vi "AuMT8852B Selected Tests.vi"(5 "Tests (All selected)":T2={"Output power (Selected)"=enum."Output power selected", "Power control (Selected)"=enum."Power control selected", "Modulation index (Selected)"=enum."Modulation index selected", "Initial carrier (Selected)"=enum."Initial carrier selected", "Carrier drift (Selected)"=enum."Carrier drift selected", "Single-slot sensitivity (Selected) "=enum."Single-slot sensitivity selected", "Multi-slot sensitivity (Selected)"=enum."Multi-slot sensitivity selected", "Maximum input power (Selected)"=enum."Maximum input power selected", "Relative transmit power (Selected)"=enum."Rel. transmit power selected", "Carrier frequency stability and modulation (Selected)"=enum."Carrier freq. and stability selected", "Differential phase encoding"=enum."Differential phase selected", "Sensitivity (Selected)"=enum."Sensitivity selected", "BER floor sensitivity (Selected)"=enum."BER floor sensitivity selected", "EDR Maximum input power (Selected)"=enum."EDR Max input power selected"}, 7 "Set/Get (Set)":enum16{"Set", "Get"}(ring), 8 "error in (no error)":errorcluster, 10 "Script (3)":i32=3, 11 "VISA session":refnum<visa-resource-name>) -> (0 "error out":errorcluster, 2 "error code":i32, 3 "VISA session out":refnum<visa-resource-name>, 4 "Tests out":T1={"Output power"=enum."Output power selected", "Power control"=enum."Power control selected", "Modulation index"=enum."Modulation index selected", "Initial carrier"=enum."Initial carrier selected", "Carrier drift"=enum."Carrier drift selected", "Single-slot sensitivity"=enum."Single-slot sensitivity selected", "Multi-slot sensitivity "=enum."Multi-slot sensitivity selected", "Maximum input iower"=enum."Maximum input power selected", "Relative transmit power (Selected)"=enum."Rel. transmit power selected", "Carrier frequency stability and modulation (Selected)"=enum."Carrier freq. and stability selected", "Differential phase encoding"=enum."Differential phase selected", "Sensitivity (Selected)"=enum."Sensitivity selected", "BER floor sensitivity (Selected)"=enum."BER floor sensitivity selected", "EDR Maximum input power (Selected)"=enum."EDR Max input power selected"})   [LabVIEW 2017]
doc: "Anritsu MT8852B Bluetooth Tester\n\nINPUTS\nSet/Get - whether the configuration is being sent to or retrieved from the instrument.\nTests - which tests are selected for the specified script.\n\nOUTPUTS\nTests Out - the present tests selected for the script."
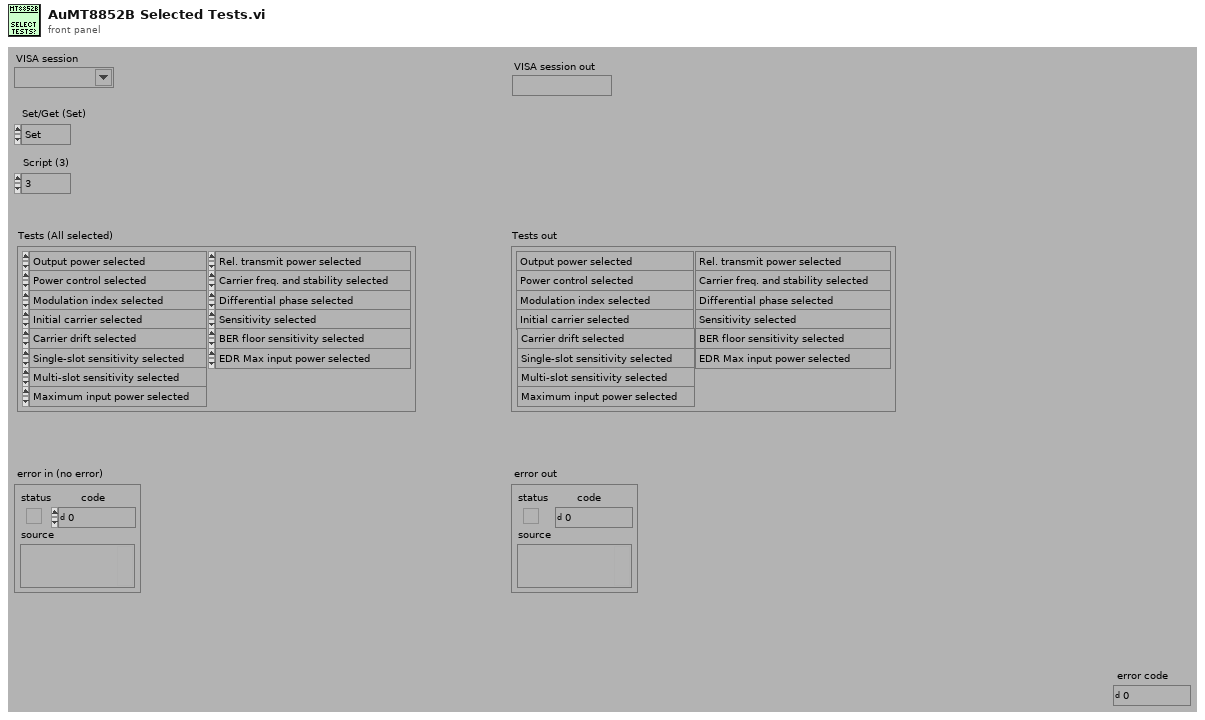
[diagram p1: front panel]
types:
  T1 = cluster{"Output power":enum16{"Output power not selected", "Output power selected"}, "Power control":enum16{"Power control not selected", "Power control selected"}, "Modulation index":enum16{"Modulation index not selected", "Modulation index selected"}, "Initial carrier":enum16{"Initial carrier not selected", "Initial carrier selected"}, "Carrier drift":enum16{"Carrier drift not selected", "Carrier drift selected"}, "Single-slot sensitivity":enum16{"Single-slot sensitivity not selected", "Single-slot sensitivity selected"}, "Multi-slot sensitivity ":enum16{"Multi-slot sensitivity not selected", "Multi-slot sensitivity selected"}, "Maximum input iower":enum16{"Maximum input power not selected", "Maximum input power selected"}, "Relative transmit power (Selected)":enum16{"Rel. transmit power not selected", "Rel. transmit power selected"}, "Carrier frequency stability and modulation (Selected)":enum16{"Carrier freq. and stability not selected", "Carrier freq. and stability selected"}, "Differential phase encoding":enum16{"Differential phase not selected", "Differential phase selected"}, "Sensitivity (Selected)":enum16{"Sensitivity not selected", "Sensitivity selected"}, "BER floor sensitivity (Selected)":enum16{"BER floor sensitivity not selected", "BER floor sensitivity selected"}, "EDR Maximum input power (Selected)":enum16{"EDR Max input power not selected", "EDR Max input power selected"}}
  T2 = cluster{"Output power (Selected)":enum16{"Output power not selected", "Output power selected"}, "Power control (Selected)":enum16{"Power control not selected", "Power control selected"}, "Modulation index (Selected)":enum16{"Modulation index not selected", "Modulation index selected"}, "Initial carrier (Selected)":enum16{"Initial carrier not selected", "Initial carrier selected"}, "Carrier drift (Selected)":enum16{"Carrier drift not selected", "Carrier drift selected"}, "Single-slot sensitivity (Selected) ":enum16{"Single-slot sensitivity not selected", "Single-slot sensitivity selected"}, "Multi-slot sensitivity (Selected)":enum16{"Multi-slot sensitivity not selected", "Multi-slot sensitivity selected"}, "Maximum input power (Selected)":enum16{"Maximum input power not selected", "Maximum input power selected"}, "Relative transmit power (Selected)":enum16{"Rel. transmit power not selected", "Rel. transmit power selected"}, "Carrier frequency stability and modulation (Selected)":enum16{"Carrier freq. and stability not selected", "Carrier freq. and stability selected"}, "Differential phase encoding":enum16{"Differential phase not selected", "Differential phase selected"}, "Sensitivity (Selected)":enum16{"Sensitivity not selected", "Sensitivity selected"}, "BER floor sensitivity (Selected)":enum16{"BER floor sensitivity not selected", "BER floor sensitivity selected"}, "EDR Maximum input power (Selected)":enum16{"EDR Max input power not selected", "EDR Max input power selected"}}
  T3 = enum16{"Simulate", "Range check", "Cache", "Query instrument status"}
  T4 = enum16{"Output power not selected", "Output power selected"}
  T5 = enum16{"Power control not selected", "Power control selected"}
  T6 = enum16{"Modulation index not selected", "Modulation index selected"}
  T7 = enum16{"Initial carrier not selected", "Initial carrier selected"}
  T8 = enum16{"Carrier drift not selected", "Carrier drift selected"}
  T9 = enum16{"Single-slot sensitivity not selected", "Single-slot sensitivity selected"}
  T10 = enum16{"Multi-slot sensitivity not selected", "Multi-slot sensitivity selected"}
  T11 = enum16{"Maximum input power not selected", "Maximum input power selected"}
  T12 = enum16{"Rel. transmit power not selected", "Rel. transmit power selected"}
  T13 = enum16{"Carrier freq. and stability not selected", "Carrier freq. and stability selected"}
  T14 = enum16{"Differential phase not selected", "Differential phase selected"}
  T15 = enum16{"Sensitivity not selected", "Sensitivity selected"}
  T16 = enum16{"BER floor sensitivity not selected", "BER floor sensitivity selected"}
  T17 = enum16{"EDR Max input power not selected", "EDR Max input power selected"}
  T18 = cluster{"[0]":i16, "[1]":i16, "[2]":i16, "[3]":i16, "[4]":i16, "[5]":i16, "[6]":i16, "[7]":i16, "[8]":i16, "[9]":i16, "[10]":i16, "[11]":i16, "[12]":i16, "[13]":i16}
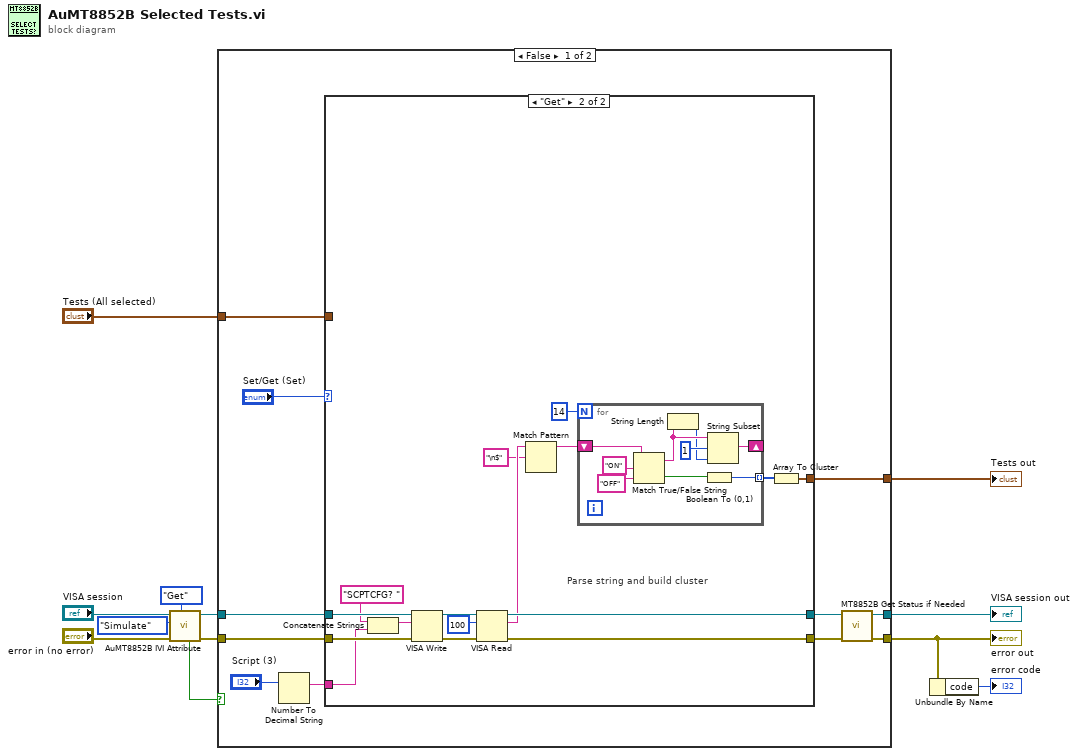
[diagram p0: block diagram]
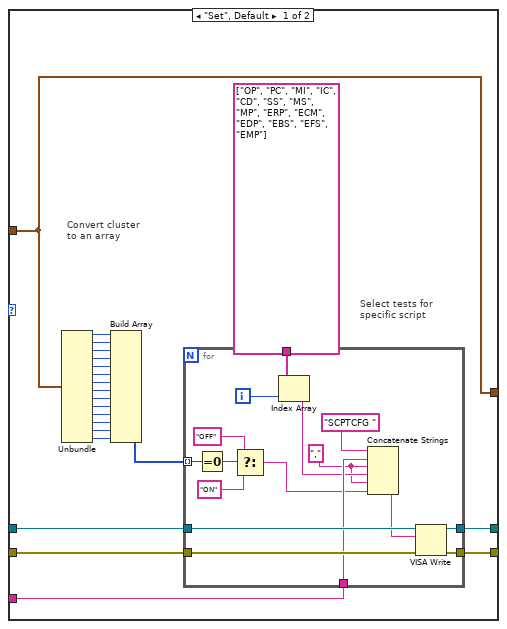
[diagram p2: hidden frame]
diagram:
  n1 = call <instrlib>:"AuMT8852B IVI Attribute.vi"("Set/Get (Set)"=enum16{"Set", "Get"}."Get", "error in (no error)"="error in (no error)", "Flag (Simulate)"=T3."Simulate", "VISA session"="VISA session") -> ("error out"=w6:errorcluster, "VISA session out"=w7:refnum<visa-resource-name>, "Value out"=w5:bool)  [unwired: 5 in]
  n2 = case shown="False" w5 {
    tunnel: [w22 w87] -> w1
    tunnel: [w21 w88] -> w12
    tunnel: w6 -> [w18 w87]
    tunnel: w7 -> [w17 w88]
    tunnel: "Tests (All selected)" -> [w16 w89]
    tunnel: [w15 w89] -> w10
    frame False {
      n3 = Number To Decimal String(number="Script (3)") -> (decimal integer string=w13:string)  [unwired: 1 in]
      n4 = case shown="\"Get\"" "Set/Get (Set)" {
        tunnel: [w42 w72] -> w19
        tunnel: w16 -> [w30 _]
        tunnel: w13 -> [w41 w66]
        tunnel: [w43 w71] -> w20
        tunnel: w17 -> [w45 w77]
        tunnel: w18 -> [w44 w76]
        tunnel: [w30 w69] -> w15
        frame "Set", Default {
          # "Select tests for \nspecific script"
          # "Convert cluster \nto an array"
          n5 = Unbundle(w30) -> ("Output power (Selected)"=w32:T4, "Power control (Selected)"=w31:T5, "Modulation index (Selected)"=w40:T6, "Initial carrier (Selected)"=w39:T7, "Carrier drift (Selected)"=w38:T8, "Single-slot sensitivity (Selected)"=w37:T9, "Multi-slot sensitivity (Selected)"=w36:T10, "Maximum input power (Selected)"=w35:T11, "Relative transmit power (Selected)"=w24:T12, "Carrier frequency stability and modulation (Selected)"=w25:T13, "Differential phase encoding"=w26:T14, "Sensitivity (Selected)"=w27:T15, "BER floor sensitivity (Selected)"=w28:T16, "EDR Maximum input power (Selected)"=w29:T17)
          n6 = Build Array(w32, w31, w40, w39, w38, w37, w36, w35, w24, w25, w26, w27, w28, w29) -> (w33:u16[])
          n7 = for {
            tunnel: w45 -> [w61]
            tunnel: w44 -> [w60]
            tunnel: [w57] -> w43
            tunnel: [w56] -> w42
            tunnel: w41 -> [w55]
            tunnel: w33 -> [w53] mode=indexing
            tunnel: string[] ["OP", "PC", "MI", "IC", "CD", "SS", "MS", "MP", "ERP", "ECM", "EDP", "EBS", "EFS", "EMP"] ("Array Constant") -> [w50]
            i -> [w49]
            w47 = "," ("Substring")
            n8 = Equal To 0?(x=w53) -> (x = 0?=w54:bool)
            n9 = Select(t="OFF", s=w54, f="ON") -> (s? t:f=w46:string)
            n10 = Index Array(array=w50, index=w49) -> (element=w48:string)
            n11 = Concatenate Strings("SCPTCFG " ("Substring"), w55, w47, w48, w47, w46) -> (w59:string)
            n12 = VISA Write(VISA resource name=w61, write buffer=w59, error in (no error)=w60) -> (VISA resource name out=w57:refnum<visa-resource-name>, error out=w56:errorcluster)  [unwired: 1 out]
          }
        }
        frame "Get" {
          # "Parse string and build cluster"
          n13 = Concatenate Strings("SCPTCFG? " ("write buffer (\"\")"), w66) -> (w67:string)
          n14 = VISA Write(VISA resource name=w77, write buffer=w67, error in (no error)=w76) -> (VISA resource name out=w75:refnum<visa-resource-name>, error out=w73:errorcluster)  [unwired: 1 out]
          n15 = VISA Read(VISA resource name=w75, byte count=u32 100 ("byte count (0)"), error in (no error)=w73) -> (VISA resource name out=w71:refnum<visa-resource-name>, read buffer=w64:string, error out=w72:errorcluster)  [unwired: 1 out]
          n16 = Match Pattern(string=w64, regular expression="\n$") -> (before substring=w63:string)  [unwired: 1 in, 3 out]
          n17 = for {
            N: 14 -> [_]
            tunnel: [w83] -> w70 mode=indexing
            shift-right: [w80] -> _
            shift-left: w63 -> [w82]
            n18 = Match True/False String(2:"OFF" ("false string"), 3:"ON" ("true string"), 4:w82) -> (0:w84:bool, 1:w79:string)
            n19 = String Length(string=w79) -> (length=w78:i32)
            n20 = Boolean To (0,1)(Boolean=w84) -> (0, 1=w83:i16)
            n21 = String Subset(string=w79, offset (0)=1, length (rest)=w78) -> (substring=w80:string)
          }
          n22 = Array To Cluster(array=w70) -> (cluster=w69:T18)
        }
      }
      n23 = call <instrlib>:"MT8852B Get Status if Needed.vi"("error in (no error)"=w19, "VISA session"=w20) -> ("error out"=w22:errorcluster, "VISA session out"=w21:refnum<visa-resource-name>)  [unwired: 8 in]
    }
    frame True {
    }
  }
  "error out" <- w1
  "VISA session out" <- w12
  "Tests out" <- w10
  n24 = Unbundle By Name(w1) -> ("code"=→"error code":i32)
